vi "REINITIALIZE INVOKE.vi"(8 "error in (no error)":errorcluster, 10 "Str Refnum":refnum<vi>, 11 "ComboBox in":refnum<vi>) -> (0 "error out":errorcluster)   [LabVIEW 2018]
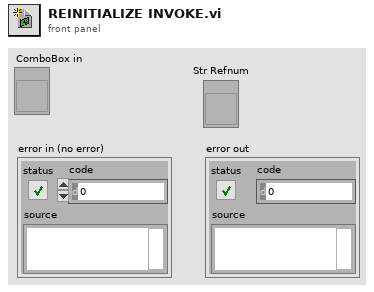
[diagram p1: front panel]
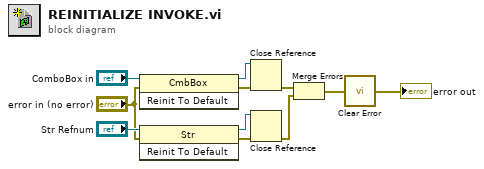
[diagram p0: block diagram]
diagram:
  n1 = invoke class="CmbBox" method="Reinit To Default"(reference="ComboBox in", error in="error in (no error)") -> (reference out=w10:refnum<vi>, error out=w9:errorcluster)  [unwired: 1 in, 1 out]
  n2 = invoke class="Str" method="Reinit To Default"(reference="Str Refnum", error in="error in (no error)") -> (reference out=w6:refnum<vi>, error out=w5:errorcluster)  [unwired: 1 in, 1 out]
  n3 = Close Reference(reference=w10, error in (no error)=w9) -> (error out=w4:errorcluster)
  n4 = Close Reference(reference=w6, error in (no error)=w5) -> (error out=w3:errorcluster)
  n5 = Merge Errors(w4, w3) -> (w2:errorcluster)
  n6 = call "Clear Error.vi"("error in"=w2) -> ("error out"=→"error out":errorcluster)
